vi "Init Event Handler.vi"(8 "error in (no error)":errorcluster, 11 "VolatusCore in":refnum<class "VolatusCore.lvclass">) -> (0 "error out":errorcluster, 3 "VolatusCore out":refnum<class "VolatusCore.lvclass">)   [LabVIEW 2020, in "Volatus.lvlib" / "VolatusCore.lvclass"]
uses:
  VolatusCore.lvclass
  VolatusCore.lvclass/VolatusCore.ctl
  <vilib>/ActorFramework/Actor/Actor.lvclass
  Event API/EventAPI.lvclass
  EventHandlerTask/EventHandlerTask.lvclass
  App/App.lvclass
  C:/Program Files (x86)/National Instruments/LabVIEW 2020/vi.lib/ActorFramework/Actor/Actor.lvclass
  C:/dev/lv20CE/relink/lv-volatus/Volatus/EventHandlerTask/EventHandlerTask.lvclass
  C:/dev/lv20CE/relink/lv-volatus/Volatus/EventHandler/EventHandler.lvclass
  C:/dev/lv20CE/relink/lv-volatus/Volatus/Event API/EventAPI.lvclass
  C:/dev/lv20CE/relink/lv-volatus/Volatus/API/API.lvclass
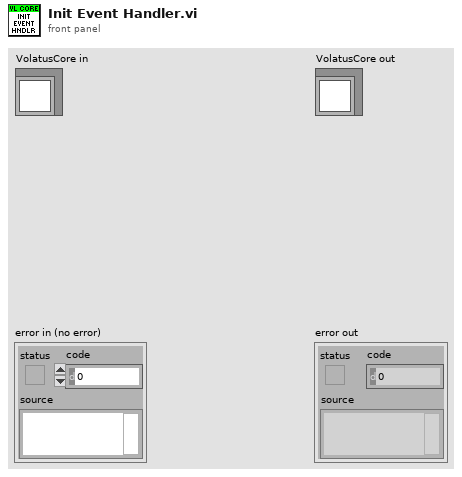
[diagram p1: front panel]
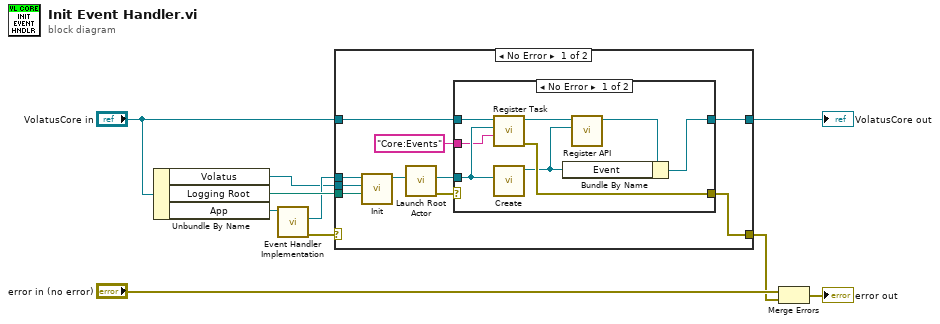
[diagram p0: block diagram]
diagram:
  n1 = Unbundle By Name("VolatusCore in") -> ("Volatus"=w1:refnum<class "VolatusAPI.lvclass">, "Logging Root"=w7:path, "App"=w9:refnum<class "App.lvclass">)
  n2 = call-dynamic "Event Handler Implementation.vi"("App in"=w9) -> ("error out"=w8:errorcluster, "EventHandlerTask"=w6:refnum<class "EventHandlerTask.lvclass">)  [unwired: 8 in, 1 out]
  n3 = case shown="No Error" w8 {
    selector: w8 -> [_ w31]
    tunnel: w6 -> [w15 _]
    tunnel: w7 -> [w14 _]
    tunnel: "VolatusCore in" -> [w18 w32]
    tunnel: [w17 w32] -> w4
    tunnel: [w16 w31] -> w2
    tunnel: w1 -> [w13 _]
    frame No Error {
      n4 = call "Init.vi"("Logging Root"=w14, "VolatusAPI"=w13, "EventHandlerTask in"=w15) -> ("EventHandlerTask out"=w12:refnum<class "EventHandlerTask.lvclass">)  [unwired: 7 in, 1 out]
      n5 = call <vilib>:"Launch Root Actor.vi"("Actor"=w12) -> ("error out"=w19:errorcluster, "Actor's Enqueuer"=w20:refnum<class "Message Enqueuer.lvclass">)  [unwired: 9 in]
      n6 = case shown="No Error" w19 {
        selector: w19 -> [_ w29]
        tunnel: w20 -> [w26 _]
        tunnel: "Core:Events" ("Task ID") -> [w25 _]
        tunnel: w18 -> [w27 w30]
        tunnel: [w22 w30] -> w17
        tunnel: [w28 w29] -> w16
        frame No Error {
          n7 = call "Register Task.vi"("Task ID"=w25, "EnQr"=w26, "VolatusCore in"=w27) -> ("error out"=w28:errorcluster, "VolatusCore out"=w23:refnum<class "VolatusCore.lvclass">)  [unwired: 7 in]
          n8 = call "Create.vi"("EnQr"=w26) -> ("Event API out"=w24:refnum<class "EventAPI.lvclass">)  [unwired: 9 in, 1 out]
          n9 = call "Register API.vi"("API"=w24, "VolatusCore in"=w23) -> ("VolatusCore out"=w21:refnum<class "VolatusCore.lvclass">)  [unwired: 8 in, 1 out]
          n10 = Bundle By Name(cluster=w21, "Event"=w24) -> (w22:refnum<class "VolatusCore.lvclass">)
        }
        frame Error {
        }
      }
    }
    frame Error {
    }
  }
  "VolatusCore out" <- w4
  n11 = Merge Errors("error in (no error)", w2) -> (→"error out":errorcluster)
